vi "GetComboBoxColumns.vi"(0 "reference in":refnum<class "DataGridView.lvclass">, 11 "error in (no error)":errorcluster) -> (4 "reference out":refnum<class "DataGridView.lvclass">, 6 "ComboBoxColumns":refnum<k24>[](array[refnum]), 15 "error out":errorcluster)   [LabVIEW 2018, in "DataGridView.lvclass"]
uses:
  DataGridView.lvclass
  System.Windows.Forms
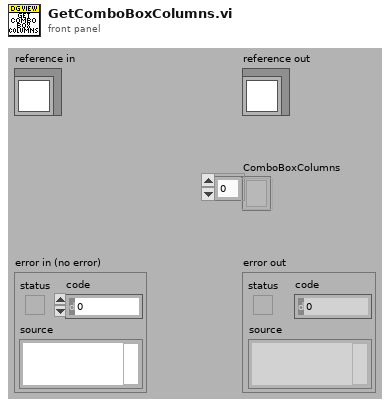
[diagram p1: front panel]
types:
  T1 = typedef "DataGridView.lvclass/ObjectAttributes.ctl" = cluster{"DataGridView":refnum<k24>, "SelectionChangedEvent":refnum<user-event>, "SelectionChanged callback ref":refnum<k27>, "LastSelectedRowIndex":i32}
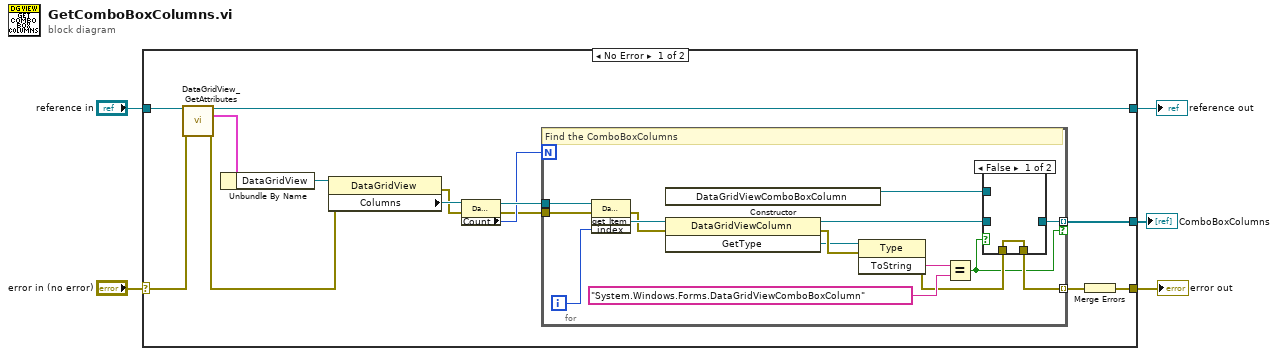
[diagram p0: block diagram]
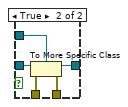
[diagram p2: hidden frame]
diagram:
  n1 = case shown="No Error" "error in (no error)" {
    selector: "error in (no error)" -> [w19 w42]
    tunnel: [w8 w42] -> w4
    tunnel: [w16 w41] -> w2
    tunnel: "reference in" -> [w17 w41]
    tunnel: [w6 _] -> w1
    frame No Error {
      n2 = call "DataGridView_GetAttributes.vi"("reference in"=w17, "error in (no error)"=w19) -> ("reference out"=w16:refnum<class "DataGridView.lvclass">, "Data"=w18:T1, "error out"=w9:errorcluster)  [unwired: 10 in, 1 out]
      n3 = Unbundle By Name(w18) -> ("DataGridView"=w10:refnum<k24>)
      n4 = property class="DataGridView"(reference=w10, error in=w9) -> (error out=w12:errorcluster, "Columns"=w15:refnum<k24>)  [unwired: 1 out]
      n5 = property class="DataGridViewColumnCollection"(reference=w15, error in=w12) -> (reference out=w14:refnum<k24>, error out=w11:errorcluster, "Count"=w13:i32)
      n6 = for {
        N: w13 -> [_]
        tunnel: w14 -> [w34]
        tunnel: w11 -> [w32]
        tunnel: [w29] -> w6 mode=indexing if=w22
        tunnel: [w27] -> w7 mode=indexing
        i -> [w33]
        # "Find the ComboBoxColumns"
        n7 = invoke class="DataGridViewColumnCollection" method="get_Item"(reference=w34, error in=w32, "index"=w33) -> (error out=w24:errorcluster, "get_Item"=w26:refnum<k24>)  [unwired: 1 in, 2 out]
        n8 = constructor class="DataGridViewComboBoxColumn"() -> (reference out=w21:refnum<k24>)  [unwired: 3 in, 2 out]
        n9 = invoke class="DataGridViewColumn" method="GetType"(reference=w26, error in=w24) -> (reference out=w25:refnum<k24>, error out=w23:errorcluster, "GetType"=w20:refnum<k24>)  [unwired: 1 in]
        n10 = invoke class="Type" method="ToString"(reference=w20, error in=w23) -> (error out=w28:errorcluster, "ToString"=w30:string)  [unwired: 1 in, 1 out]
        n11 = Equal?(x=w30, y="System.Windows.Forms.DataGridViewComboBoxColumn") -> (x = y?=w22:bool)
        n12 = case shown="False" w22 {
          tunnel: [_ w40] -> w29
          tunnel: w21 -> [_ w39]
          tunnel: w28 -> [w35 w38]
          tunnel: [w35 w37] -> w27
          tunnel: w25 -> [_ w36]
          frame False {
          }
          frame True {
            n13 = To More Specific Class(target class=w39, reference=w36, error in=w38) -> (specific class reference=w40:refnum<k24>, error out=w37:errorcluster)
          }
        }
      }
      n14 = Merge Errors(w7) -> (w8:errorcluster)
    }
    frame Error {
    }
  }
  "error out" <- w4
  "reference out" <- w2
  "ComboBoxColumns" <- w1
